vi "Deadband Joystick.vi"(1 "Axes":dbl[](array[numeric])) -> (0 "Axes":dbl[](array[numeric]))   [LabVIEW 2018]
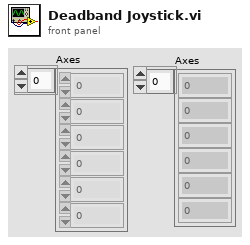
[diagram p1: front panel]
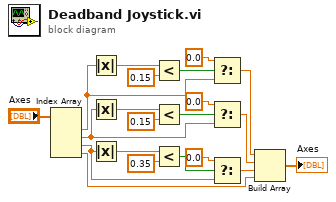
[diagram p0: block diagram]
diagram:
  n1 = Index Array(array="Axes") -> (element #1=w6:dbl, element #2=w4:dbl, element #3=w1:dbl, element #4=w20:dbl)  [unwired: 4 in]
  n2 = Absolute Value(x=w6) -> (abs(x)=w14:dbl)
  n3 = Absolute Value(x=w4) -> (abs(x)=w10:dbl)
  n4 = Absolute Value(x=w1) -> (abs(x)=w18:dbl)
  n5 = Less?(x=w14, y=0.15) -> (x < y?=w11:bool)
  n6 = Less?(x=w10, y=0.15) -> (x < y?=w7:bool)
  n7 = Less?(x=w18, y=0.35) -> (x < y?=w15:bool)
  n8 = Select(t=0.0, s=w11, f=w6) -> (s? t:f=w5:dbl)
  n9 = Select(t=0.0, s=w7, f=w4) -> (s? t:f=w3:dbl)
  n10 = Select(t=0.0, s=w15, f=w1) -> (s? t:f=w2:dbl)
  n11 = Build Array(w5, w3, w2, w20) -> (→"Axes":dbl[])
